vi "QD_DAQ.vi"(0 "State_and_Data_In":T1, 1 "Max_Queue_Size_In":i32=-1, 2 "Queue_Name_In":string, 5 "Data_In_N":T1[](array[typedef]), 7 "Time_Out_In_ms (-1)":i32, 11 "Error_In":errorcluster, 13 "Queue_Operation":T2=enum."Enqueue") -> (4 "State_and_Data_Out":T1, 15 "Error_Out":errorcluster)   [LabVIEW 2021]
doc: "Used to send the State and event data between loops and VIs"
uses:
  Controls/State_and_Data.ctl
  Controls/Error_Data.ctl
  Controls/Queue_Operation_Select.ctl
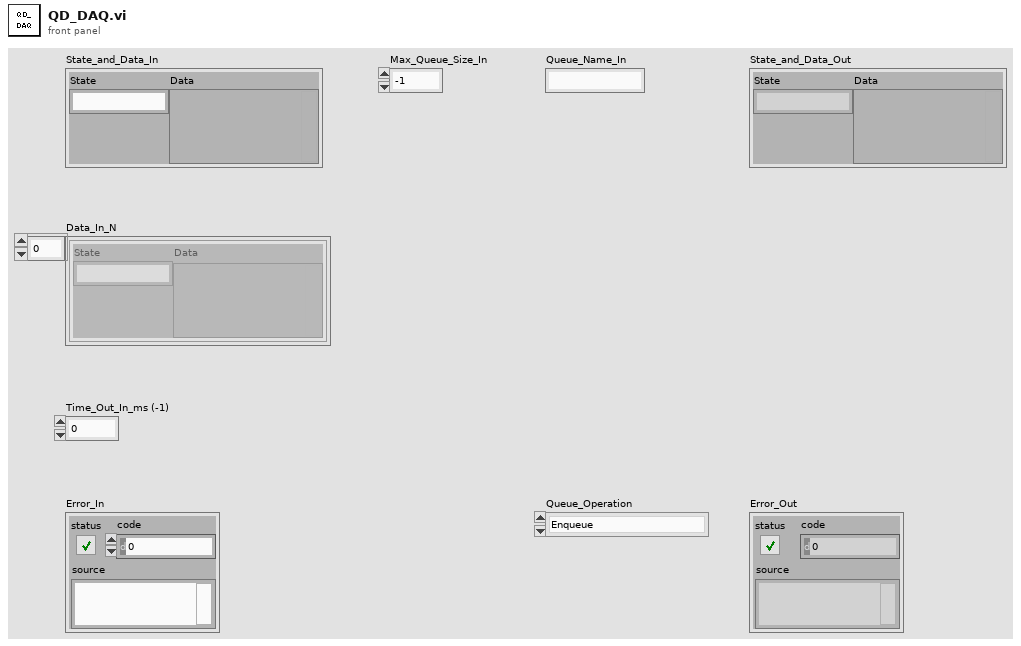
[diagram p1: front panel]
types:
  T1 = typedef "State_and_Data.ctl" = cluster{"State":string, "Data":variant}
  T2 = typedef "Queue_Operation_Select.ctl" = enum16{"Obtain_Queue", "Enqueue", "Enqueue_First", "Enqueue_N", "Lossy_Enqueue", "Preview", "Queue_Status", "Dequeue", "Flush", "Release_Queue"}
  T3 = typedef "Error_Data.ctl" = cluster{"Module_Name":string, "Error":errorcluster}
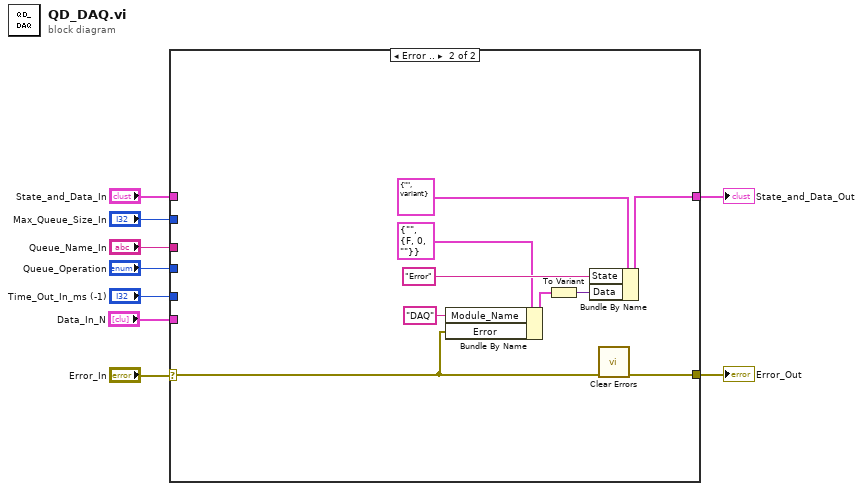
[diagram p0: block diagram]
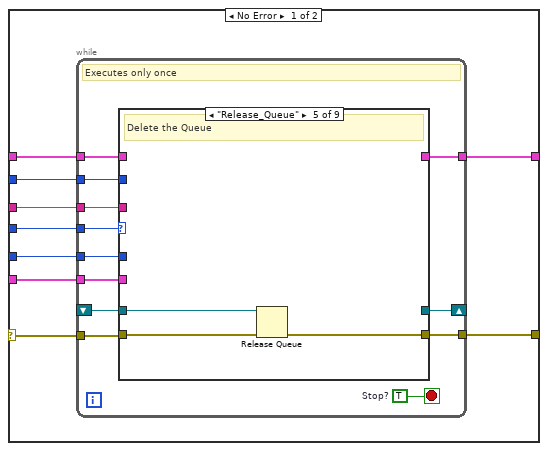
[diagram p2: hidden frame]
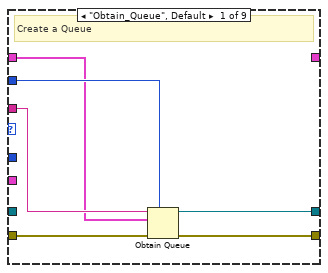
[diagram p3: hidden frame]
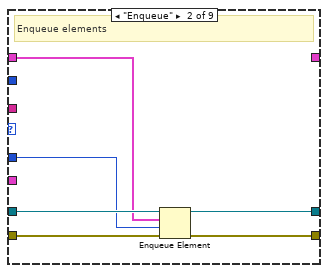
[diagram p4: hidden frame]
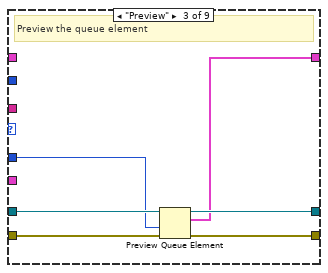
[diagram p5: hidden frame]
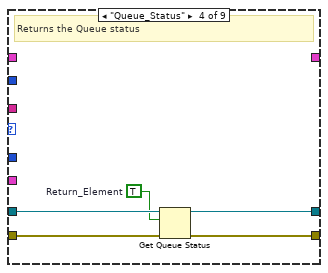
[diagram p6: hidden frame]
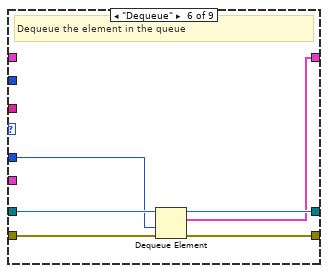
[diagram p7: hidden frame]
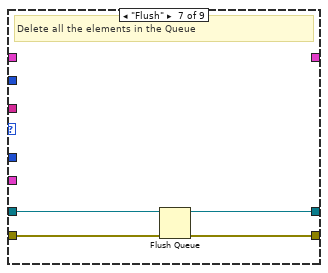
[diagram p8: hidden frame]
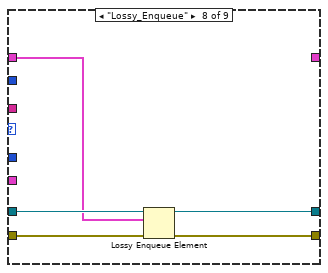
[diagram p9: hidden frame]
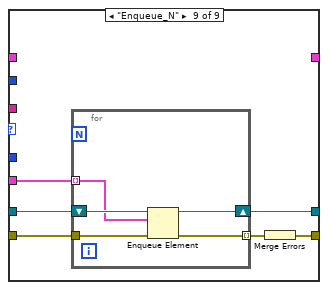
[diagram p10: hidden frame]
diagram:
  n1 = case shown="Error .." "Error_In" {
    selector: "Error_In" -> [w11 w83]
    tunnel: "Max_Queue_Size_In" -> [w18 _]
    tunnel: [w17 w86] -> w8
    tunnel: "State_and_Data_In" -> [w16 _]
    tunnel: "Time_Out_In_ms (-1)" -> [w15 _]
    tunnel: [w14 w85] -> w5
    tunnel: "Queue_Operation" -> [w13 _]
    tunnel: "Queue_Name_In" -> [w12 _]
    tunnel: "Data_In_N" -> [w10 _]
    frame No Error {
      n2 = while {
        tunnel: w18 -> [w30]
        tunnel: w15 -> [w27]
        tunnel: w13 -> [w24]
        shift-right: [w25] -> _
        shift-left: _ -> [w21]
        tunnel: w11 -> [w22]
        tunnel: [w29] -> w17
        tunnel: w16 -> [w28]
        tunnel: [w26] -> w14
        tunnel: w12 -> [w23]
        tunnel: w10 -> [w19]
        stop <- w20 stop-if-true
        w20 = TRUE  # Stop?
        # "Executes only once"
        n3 = case shown="\"Release_Queue\"" w24 {
          tunnel: w22 -> [w36 w42 w47 w52 w55 w61 w65 w70 w77]
          tunnel: w23 -> [w34 _ _ _ _ _ _ _ _]
          tunnel: w30 -> [w33 _ _ _ _ _ _ _ _]
          tunnel: [w31 w38 w46 w51 _ w60 w64 w69 w74] -> w25
          tunnel: [w35 w41 w45 w50 w54 w58 w63 w68 w73] -> w29
          tunnel: w21 -> [_ w40 w48 w53 w56 w62 w66 w71 w75]
          tunnel: w28 -> [w32 w39 _ _ _ _ _ w67 _]
          tunnel: w27 -> [_ w37 w44 _ _ w57 _ _ _]
          tunnel: [_ _ w43 _ _ w59 _ _ _] -> w26
          tunnel: w19 -> [_ _ _ _ _ _ _ _ w72]
          frame "Obtain_Queue", Default {
            # "Create a Queue"
            n4 = Obtain Queue(max queue size (-1, unlimited)=w33, name (unnamed)=w34, element data type=w32, error in (no error)=w36) -> (queue out=w31:refnum<queue>, error out=w35:errorcluster)  [unwired: 1 in, 1 out]
          }
          frame "Enqueue" {
            # "Enqueue elements"
            n5 = Enqueue Element(queue=w40, element=w39, timeout in ms (-1)=w37, error in (no error)=w42) -> (queue out=w38:refnum<queue>, error out=w41:errorcluster)  [unwired: 1 out]
          }
          frame "Preview" {
            # "Preview the queue element"
            n6 = Preview Queue Element(queue=w48, timeout in ms (-1)=w44, error in (no error)=w47) -> (queue out=w46:refnum<queue>, element=w43:T1, error out=w45:errorcluster)  [unwired: 1 out]
          }
          frame "Queue_Status" {
            w49 = TRUE  # Return_Element
            # "Returns the Queue status"
            n7 = Get Queue Status(queue=w53, return elements? (F)=w49, error in (no error)=w52) -> (queue out=w51:refnum<queue>, error out=w50:errorcluster)  [unwired: 6 out]
          }
          frame "Release_Queue" {
            # "Delete the Queue"
            n8 = Release Queue(queue=w56, error in (no error)=w55) -> (error out=w54:errorcluster)  [unwired: 1 in, 2 out]
          }
          frame "Dequeue" {
            # "Dequeue the element in the queue"
            n9 = Dequeue Element(queue=w62, timeout in ms (-1)=w57, error in (no error)=w61) -> (queue out=w60:refnum<queue>, element=w59:T1, error out=w58:errorcluster)  [unwired: 1 out]
          }
          frame "Flush" {
            # "Delete all the elements in the Queue"
            n10 = Flush Queue(queue=w66, error in (no error)=w65) -> (queue out=w64:refnum<queue>, error out=w63:errorcluster)  [unwired: 1 out]
          }
          frame "Lossy_Enqueue" {
            n11 = Lossy Enqueue Element(queue=w71, element=w67, error in (no error)=w70) -> (queue out=w69:refnum<queue>, error out=w68:errorcluster)  [unwired: 2 out]
          }
          frame "Enqueue_N" {
            n12 = for {
              tunnel: w77 -> [w82]
              tunnel: [w81] -> w76 mode=indexing
              shift-right: [w79] -> w74
              shift-left: w75 -> [w80]
              tunnel: w72 -> [w78] mode=indexing
              n13 = Enqueue Element(queue=w80, element=w78, error in (no error)=w82) -> (queue out=w79:refnum<queue>, error out=w81:errorcluster)  [unwired: 1 in, 1 out]
            }
            n14 = Merge Errors(w76) -> (w73:errorcluster)
          }
        }
      }
    }
    frame Error {
      n15 = Bundle By Name(cluster=T3 {"Module_Name"="", "Error"={"status"=FALSE, "code"=0, "source"=""}} ("Error_Data"), "Module_Name"="DAQ", "Error"=w83) -> (w84:T3)
      n16 = To Variant(anything=w84) -> (Variant=w88:variant)
      n17 = Bundle By Name(cluster=T1 {"State"="", "Data"=variant} ("State_and_Data_In"), "State"="Error", "Data"=w88) -> (w85:T1)
      n18 = call <vilib>:"Clear Errors.vi"("error in (no error)"=w83) -> ("error out"=w86:errorcluster)  [unwired: 5 in, 1 out]
    }
  }
  "Error_Out" <- w8
  "State_and_Data_Out" <- w5
